vi "例7.6利用波形图表显示单条曲线.vi"() -> ()   [LabVIEW 2017]
panel:
  out "波形图表 2":dbl[](graph)
  in  "停止":bool
  out "波形图表":dbl(graph)
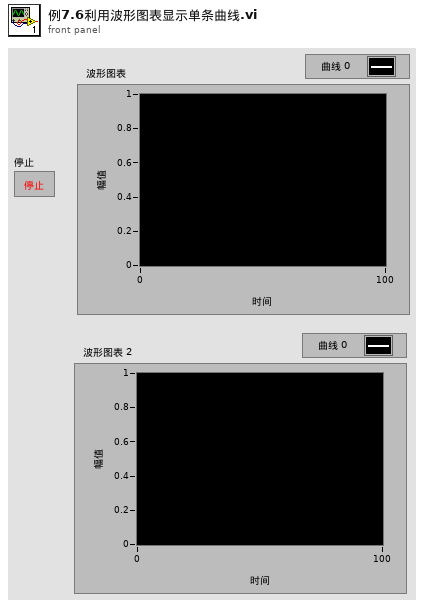
[diagram p1: front panel]
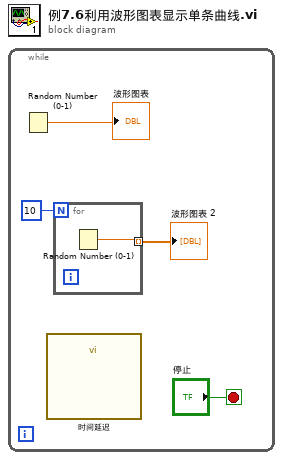
[diagram p0: block diagram]
diagram:
  n1 = while {
    stop <- "停止" stop-if-true
    n2 = Random Number (0-1)() -> (number: 0 to 1=→"波形图表":dbl)
    n3 = call "时间延迟"() -> ()  [unwired: 11 in, 1 out]
    n4 = for {
      N: 10 -> [_]
      tunnel: [w5] -> w1 mode=indexing
      n5 = Random Number (0-1)() -> (number: 0 to 1=w5:dbl)
    }
    "波形图表 2" <- w1
  }
